vi "Test 1021.vi"() -> ()   [LabVIEW 2020]
uses:
  WS1021/WS1021.lvclass
  Controls/Change setting mode enum.ctl
  PIC-device/PIC-Device.lvclass
panel:
  out "Changes":cluster{"Name":string, "Value":string}[][](array[cluster])
  in  "Stop Button":bool
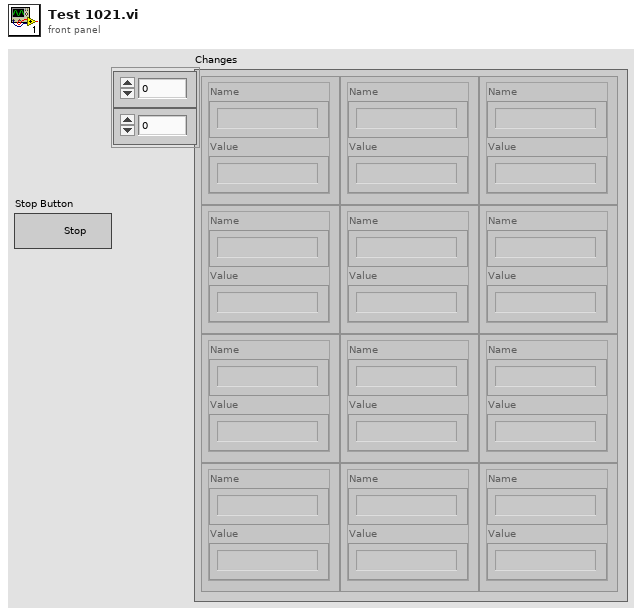
[diagram p1: front panel]
types:
  T1 = typedef "PIC-Device.lvclass/Change setting mode enum.ctl" = enum16{"Init", "Next", "Reset"}
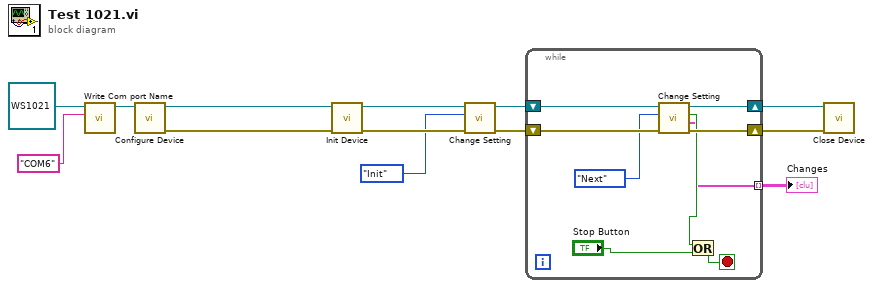
[diagram p0: block diagram]
diagram:
  n1 = call-dynamic "Write Com port Name.vi"("Com port Name"="COM6", "Device in"=refnum<class "WS1021.lvclass"> refnum ("WS1021.lvclass")) -> ("Device out"=w4:refnum<class "WS1021.lvclass">)  [unwired: 9 in]
  n2 = call-dynamic "Configure Device.vi"("WS1021 in"=w4) -> ("error out"=w13:errorcluster, "WS1021 out"=w3:refnum<class "WS1021.lvclass">)  [unwired: 9 in]
  n3 = call-dynamic "Init Device.vi"("error in (no error)"=w13, "Toggle 8 in"=w3) -> ("error out"=w11:errorcluster, "Toggle 8 out"=w12:refnum<class "WS1021.lvclass">)  [unwired: 8 in]
  n4 = call-dynamic "Change Setting.vi"("error in (no error)"=w11, "Change setting mode"=Change_setting_mode_enum."Init", "Toggle 8 in"=w12) -> ("error out"=w6:errorcluster, "Toggle 8 out"=w9:refnum<class "WS1021.lvclass">)  [unwired: 5 in, 2 out]
  n5 = while {
    shift-right: [w21] -> w8
    shift-left: w9 -> [w22]
    shift-right: [w20] -> w7
    shift-left: w6 -> [w19]
    tunnel: [w14] -> w1 mode=indexing
    stop <- w16 stop-if-true
    n6 = call-dynamic "Change Setting.vi"("error in (no error)"=w19, "Change setting mode"=Change_setting_mode_enum."Next", "Toggle 8 in"=w22) -> ("error out"=w20:errorcluster, "Changes"=w14:cluster{"Name":string, "Value":string}[], "Last setting"=w17:bool, "Toggle 8 out"=w21:refnum<class "WS1021.lvclass">)  [unwired: 5 in]
    n7 = Or(x=w17, y="Stop Button") -> (x .or. y?=w16:bool)
  }
  "Changes" <- w1
  n8 = call-dynamic "Close Device.vi"("error in (no error)"=w7, "Device in"=w8) -> ()  [unwired: 8 in, 2 out]
